vi "Destroy User Event - Stop.vi"(8 "에러 입력(에러 없음)":errorcluster, 11 "사용자 이벤트 입력":refnum<user-event>) -> (0 "에러 출력":errorcluster)   [LabVIEW 2020]
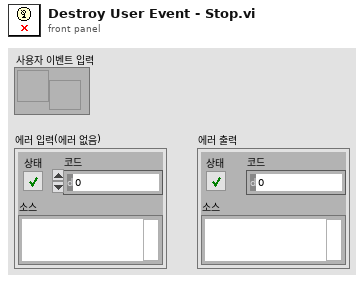
[diagram p1: front panel]
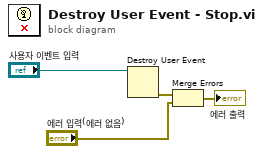
[diagram p0: block diagram]
diagram:
  n1 = Destroy User Event(user event="사용자 이벤트 입력") -> (error out=w3:errorcluster)  [unwired: 1 in]
  n2 = Merge Errors(w3, "에러 입력(에러 없음)") -> (→"에러 출력":errorcluster)
